vi "ConfigureDlg.vi"(8 "error in (no error)":errorcluster, 11 "PmuTestFunctions in":refnum<class "PmuTestFunctions.lvclass">) -> (0 "error out":errorcluster, 2 "Changed":bool, 3 "PmuTestFunctions out":refnum<class "PmuTestFunctions.lvclass">)   [LabVIEW 2018, in "Functions.lvlib" / "PmuTestFunctions.lvclass"]
uses:
  PmuTestFunctions.lvclass
  X:/Projects/PMUCal/Modules/FGen/MemberClasses/ArbitraryFunction/ArbitraryFunction.lvclass
  X:/Projects/PMUCal/Modules/FGen/MemberClasses/FunctionBaseClass/FunctionBase.lvclass
  ArbitraryFunction/TypeDefs/Arbs.ctl
  Typedefs/PmuTestParams.ctl
  ArbitraryFunction/ArbitraryFunction.lvclass/ArbitraryFunction.ctl
  PmuTestFunctions.lvclass/PmuTestFunctions.ctl
  FunctionBaseClass/FunctionBase.lvclass/FunctionBase.ctl
  ArbitraryFunction/TypeDefs/Arbitrary.ctl
  ArbitraryFunction/Accessors/Read SampleRate.vi
  Accessors/Read PmuTestParams.vi
  Accessors/Read T0.vi
  ArbitraryFunction/Accessors/Read Arbs.vi
  Accessors/Read SettlingTime.vi
  FunctionBaseClass/Accessors/Read FunctionIniFilePath.vi
  ArbitraryFunction/Accessors/Write SampleRate.vi
  Accessors/Write PmuTestParams.vi
  ArbitraryFunction/Accessors/Write Arbs.vi
  ArbitraryFunction/Accessors/Write Count.vi
  Accessors/Write SettlingTime.vi
  FunctionBaseClass/Accessors/Write FunctionIniFilePath.vi
  <vilib>/Utility/config.llb/NI_LVConfig.lvlib
  ArbitraryFunction/ArbitraryFunction.lvclass
panel:
  in  "btnSaveAs":bool
  in  "SettlingTime":dbl
  in  "T0":dbl
  in  "btnSave":bool
  in  "btnCancel":bool
  in  "SampleRate":dbl
  in  "PmuTestParams":T1
  in  "ARBS":T2[](array[typedef])
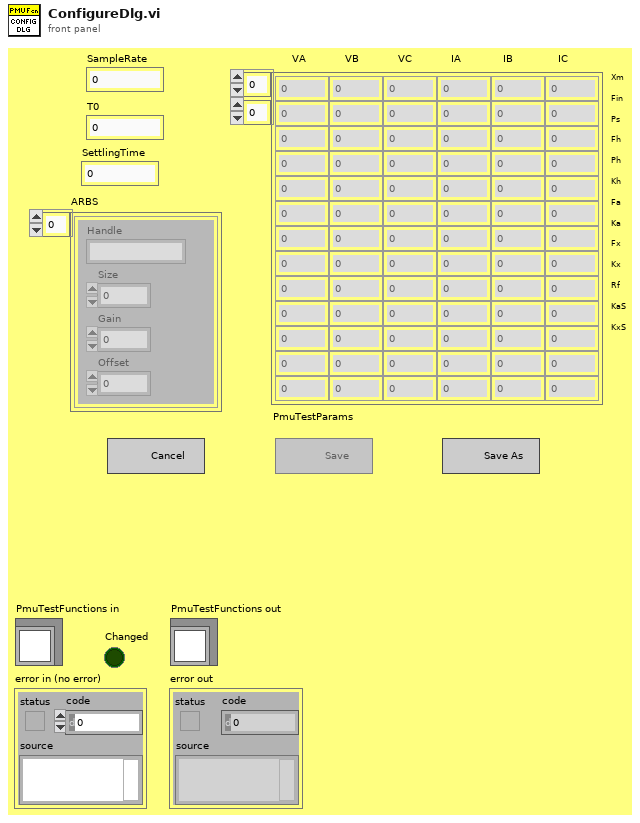
[diagram p1: front panel]
types:
  T1 = typedef "Functions.lvlib/PmuTestFunctions.lvclass/PmuTestParams.ctl" = dbl[][]
  T2 = typedef "Functions.lvlib/ArbitraryFunction.lvclass/Arbs.ctl" = cluster{"Handle":string, "Size":i32, "Gain":dbl, "Offset":dbl}
  T3 = enum32{"Invalid", "Standard", "Closed", "Hidden", "Minimized", "Maximized"}
  T4 = enum32{"Invalid", "Default", "Floating", "Floating/Auto-Hide", "Modal"}
  T5 = enum8{"Enabled", "Disabled", "Disabled and Grayed Out"}
  T6 = cluster{"Handle":string, "Size":i32, "Gain":dbl, "Offset":dbl}
  T7 = typedef "Functions.lvlib/ArbitraryFunction.lvclass/Arbitrary.ctl" = cluster{"Handle":string, "Size":i32, "Gain":dbl, "Offset":dbl, "Waveform":waveform(dbl)}
  T8 = typedef "NI_LVConfig.lvlib/Config Data RefNum.ctl" = refnum<k1>
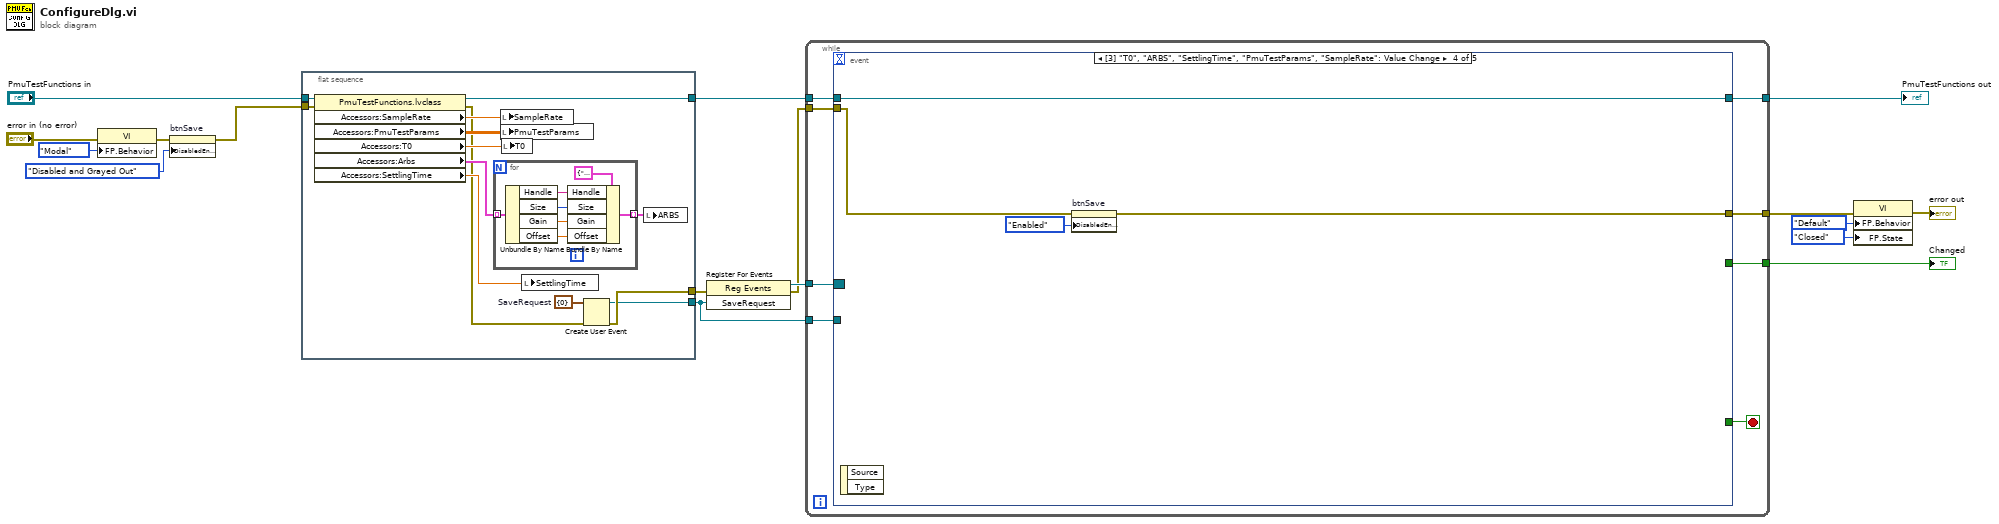
[diagram p0: block diagram]
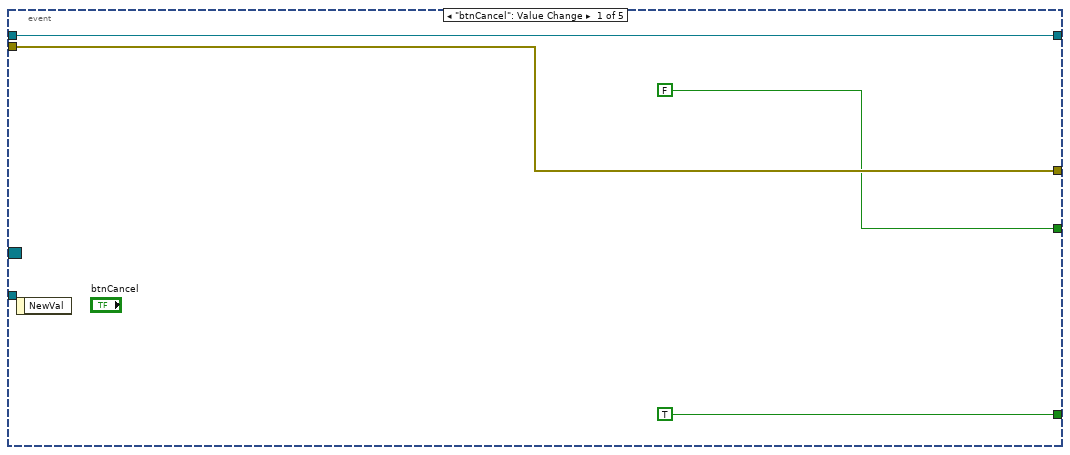
[diagram p2: hidden frame]
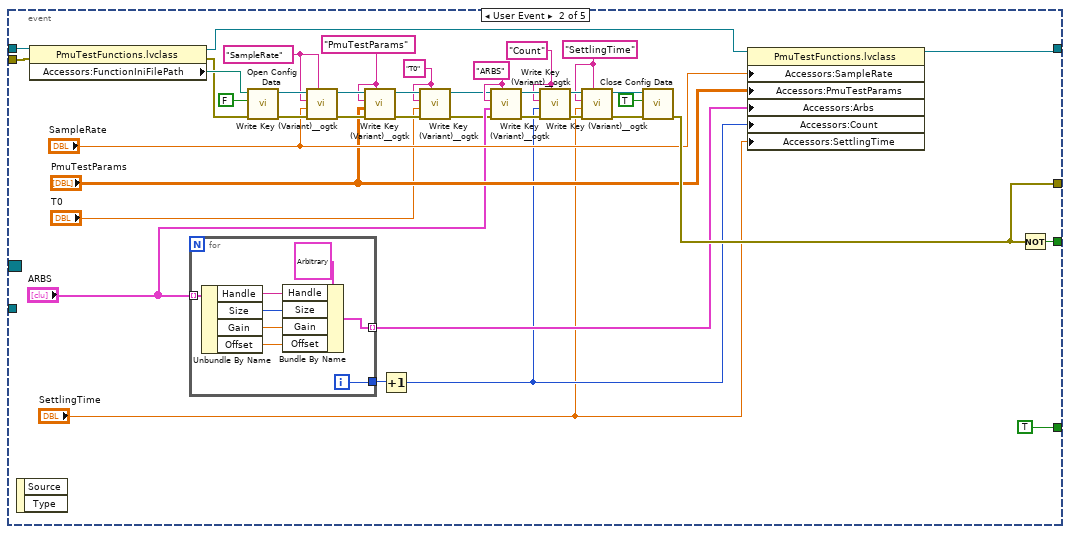
[diagram p3: hidden frame]
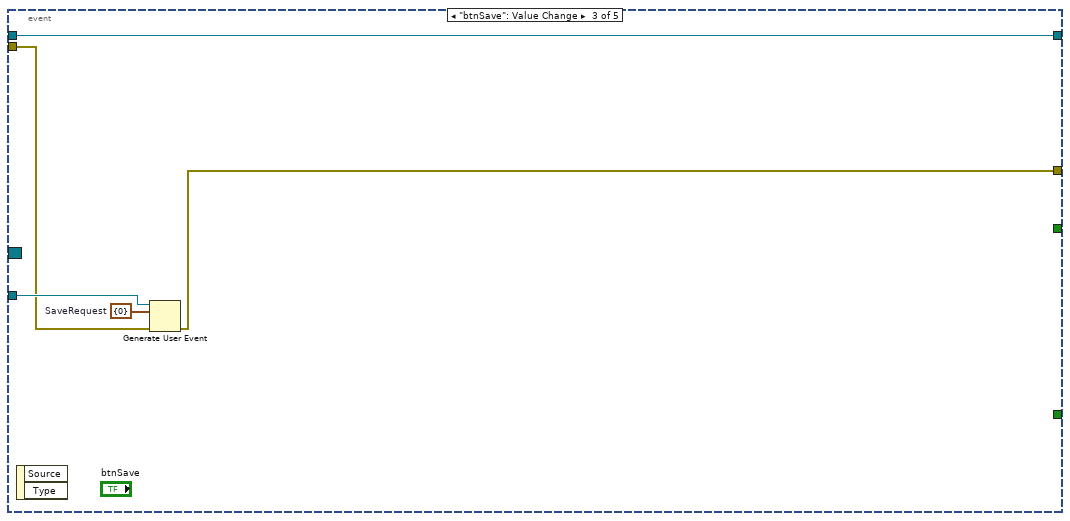
[diagram p4: hidden frame]
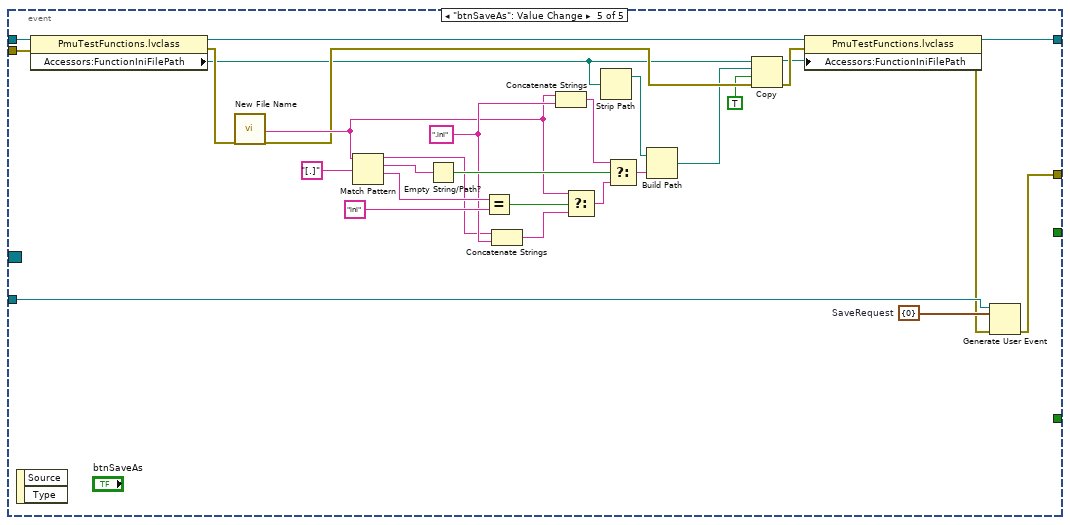
[diagram p5: hidden frame]
diagram:
  n1 = property class="VI"(error in="error in (no error)", "FP.Behavior"=T4."Modal" ("Front Panel Window:Behavior")) -> (error out=w5:errorcluster)  [unwired: 1 in, 1 out]
  n2 = property on="btnSave" class="Bool"(error in=w5, "DisabledEnum"=T5."Disabled and Grayed Out" ("Disabled")) -> (error out=w12:errorcluster)  [unwired: 1 in, 1 out]
  n3 = flat-sequence {
    tunnel: "PmuTestFunctions in" -> [w30]
    tunnel: [w29] -> w16
    tunnel: w12 -> [w27]
    tunnel: [w19] -> w11
    tunnel: [w18] -> w9
    frame #0 {
      w21 = cluster{"num":i32} {"num"=0}  # SaveRequest
      n4 = property class="PmuTestFunctions.lvclass"(reference=w30, error in=w27) -> (reference out=w29:refnum<class "PmuTestFunctions.lvclass">, error out=w20:errorcluster, "Accessors:SampleRate"=w26:dbl, "Accessors:PmuTestParams"=w25:T1, "Accessors:T0"=w24:dbl, "Accessors:Arbs"=w28:T7[], "Accessors:SettlingTime"=w22:dbl)
      n5 = for {
        tunnel: w28 -> [w37] mode=indexing
        tunnel: [w31] -> w23 mode=indexing
        n6 = Unbundle By Name(w37) -> ("Handle"=w35:string, "Size"=w34:i32, "Gain"=w33:dbl, "Offset"=w32:dbl)
        n7 = Bundle By Name(cluster=T6 {"Handle"="", "Size"=0, "Gain"=0.0, "Offset"=0.0} ("Arbs"), "Handle"=w35, "Size"=w34, "Gain"=w33, "Offset"=w32) -> (w31:T6)
      }
      n8 = local write "SampleRate"(w26) -> ()
      n9 = local write "PmuTestParams"(w25) -> ()
      n10 = local write "T0"(w24) -> ()
      n11 = local write "SettlingTime"(w22) -> ()
      n12 = Create User Event(user event datatype=w21, error in=w20) -> (user event=w18:refnum<user-event>, error out=w19:errorcluster)
      n13 = local write "ARBS"(w23) -> ()
    }
  }
  n14 = register-events(error in=w11, w9) -> (reference out=w10:refnum<event-registration>, error out=w8:errorcluster)  [unwired: 1 in]
  n15 = while {
    tunnel: w16 -> [w43]
    tunnel: w8 -> [w45]
    tunnel: [w44] -> w3
    tunnel: [w42] -> w15
    tunnel: [w41] -> w14
    tunnel: w10 -> [w39]
    tunnel: w9 -> [w38]
    stop <- w40 stop-if-true
    n16 = event shown="[3] \"T0\", \"ARBS\", \"SettlingTime\", \"PmuTestParams\", \"SampleRate\": Value Change" {
      selector: w39 -> [_ _ _ _ _]
      dyn-events: _ -> [_ _ _ _ _]
      timeout: _ -> [_ _ _ _ _]
      tunnel: [w49 w71 w98 w102 w113] -> w44
      tunnel: w45 -> [w49 w84 w99 w104 w119]
      tunnel: w43 -> [w48 w88 w97 w105 w121]
      tunnel: [w48 w65 w97 w105 w117] -> w42
      tunnel: [FALSE w72 _ _ _] -> w41
      tunnel: [TRUE TRUE _ _ _] -> w40
      tunnel: w38 -> [_ _ w100 _ w115]
      event "btnCancel": Value Change {
        n17 = event-data() -> ()  [unwired: 1 in, 1 out]
      }
      event User Event {
        w53 = "SettlingTime" ("section")
        w59 = "T0" ("section")
        w74 = "Count" ("section")
        w63 = "ARBS" ("section (optional)")
        w77 = "PmuTestParams" ("section")
        w81 = "SampleRate" ("section")
        n18 = event-data() -> ()  [unwired: 1 in, 2 out]
        n19 = property class="PmuTestFunctions.lvclass"(reference=w88, error in=w84) -> (reference out=w70:refnum<class "PmuTestFunctions.lvclass">, error out=w83:errorcluster, "Accessors:FunctionIniFilePath"=w87:path)
        n20 = for {
          tunnel: "ARBS" -> [w95] mode=indexing
          tunnel: [w90] -> w67 mode=indexing
          tunnel: [w89] -> w85
          i -> [w89]
          n21 = Unbundle By Name(w95) -> ("Handle"=w94:string, "Size"=w91:i32, "Gain"=w92:dbl, "Offset"=w93:dbl)
          n22 = Bundle By Name(cluster=T7 {"Handle"="", "Size"=0, "Gain"=0.0, "Offset"=0.0, "Waveform"={"t0"=timestamp(0 s since 1904-01-01), "dt"=1.0, "Y"=[]}} ("Arbitrary"), "Handle"=w94, "Size"=w91, "Gain"=w92, "Offset"=w93) -> (w90:T7)
        }
        n23 = call <vilib>:"Open Config Data.vi"("error in (no error)"=w83, "create file if necessary (T)"=FALSE, "configuration file path"=w87) -> ("error out"=w80:errorcluster, "refnum"=w82:T8)  [unwired: 6 in, 1 out]
        n24 = call <userlib>:"Write Key (Variant)__ogtk.vi"("section"=w81, "error in (no error)"=w80, "key-value"="SampleRate", "key (optional)"=w81, "refnum"=w82) -> ("error out"=w79:errorcluster, "refnum out"=w78:T8)  [unwired: 5 in]
        n25 = call <userlib>:"Write Key (Variant)__ogtk.vi"("section"=w77, "error in (no error)"=w79, "key-value"="PmuTestParams", "key (optional)"=w77, "refnum"=w78) -> ("error out"=w61:errorcluster, "refnum out"=w60:T8)  [unwired: 5 in]
        n26 = Increment(x=w85) -> (x+1=w66:i32)
        n27 = call <userlib>:"Write Key (Variant)__ogtk.vi"("section"=w59, "error in (no error)"=w61, "key-value"="T0", "key (optional)"=w59, "refnum"=w60) -> ("error out"=w58:errorcluster, "refnum out"=w57:T8)  [unwired: 5 in]
        n28 = call <userlib>:"Write Key (Variant)__ogtk.vi"("section"=w63, "error in (no error)"=w58, "key-value"="ARBS", "key (optional)"=w63, "refnum"=w57) -> ("error out"=w76:errorcluster, "refnum out"=w75:T8)  [unwired: 5 in]
        n29 = call <userlib>:"Write Key (Variant)__ogtk.vi"("section"=w74, "error in (no error)"=w76, "key-value"=w66, "key (optional)"=w74, "refnum"=w75) -> ("error out"=w55:errorcluster, "refnum out"=w54:T8)  [unwired: 5 in]
        n30 = call <userlib>:"Write Key (Variant)__ogtk.vi"("section"=w53, "error in (no error)"=w55, "key-value"="SettlingTime", "key (optional)"=w53, "refnum"=w54) -> ("error out"=w51:errorcluster, "refnum out"=w52:T8)  [unwired: 5 in]
        n31 = call <vilib>:"Close Config Data.vi"("error in (no error)"=w51, "write file if changed (T)"=TRUE, "refnum"=w52) -> ("error out"=w71:errorcluster)  [unwired: 7 in, 1 out]
        n32 = property class="PmuTestFunctions.lvclass"(reference=w70, "Accessors:SampleRate"="SampleRate", "Accessors:PmuTestParams"="PmuTestParams", "Accessors:Arbs"=w67, "Accessors:Count"=w66, "Accessors:SettlingTime"="SettlingTime") -> (reference out=w65:refnum<class "PmuTestFunctions.lvclass">)  [unwired: 1 in, 1 out]
        n33 = Not(x=w71) -> (.not. x?=w72:bool)
      }
      event "btnSave": Value Change {
        w101 = cluster{"num":i32} {"num"=0}  # SaveRequest
        n34 = event-data() -> ()  [unwired: 1 in, 2 out]
        n35 = Generate User Event(user event=w100, event data cluster=w101, error in=w99) -> (error out=w98:errorcluster)  [unwired: 1 in, 1 out]
      }
      event "T0", "ARBS", "SettlingTime", "SampleRate": Value Change {
        n36 = event-data() -> ()  [unwired: 1 in, 2 out]
        n37 = property on="btnSave" class="Bool"(error in=w104, "DisabledEnum"=T5."Enabled" ("Disabled")) -> (error out=w102:errorcluster)  [unwired: 1 in, 1 out]
      }
      event "btnSaveAs": Value Change {
        w116 = cluster{"num":i32} {"num"=0}  # SaveRequest
        w125 = ".ini" ("string")
        n38 = event-data() -> ()  [unwired: 1 in, 2 out]
        n39 = property class="PmuTestFunctions.lvclass"(reference=w121, error in=w119) -> (reference out=w120:refnum<class "PmuTestFunctions.lvclass">, error out=w118:errorcluster, "Accessors:FunctionIniFilePath"=w110:path)
        n40 = call "New File Name"("error in (no error)"=w118) -> ("File Name"=w122:string, "error out"=w112:errorcluster)  [unwired: 16 in, 1 out]
        n41 = Match Pattern(string=w122, regular expression="[.]" ("string")) -> (before substring=w124:string, match substring=w128:string, after substring=w127:string)  [unwired: 1 in, 1 out]
        n42 = Empty String/Path?(string/path=w128) -> (empty?=w133:bool)
        n43 = Equal?(x=w127, y="ini" ("string")) -> (x = y?=w131:bool)
        n44 = Concatenate Strings(w124, w125) -> (w123:string)
        n45 = Concatenate Strings(w122, w125) -> (w132:string)
        n46 = Select(t=w122, s=w131, f=w123) -> (s? t:f=w130:string)
        n47 = Strip Path(path=w110) -> (stripped path=w109:path)  [unwired: 1 out]
        n48 = Select(t=w132, s=w133, f=w130) -> (s? t:f=w134:string)
        n49 = Build Path(base path=w109, name or relative path=w134) -> (appended path=w107:path)
        n50 = Copy(8:w112, 9:TRUE ("overwrite (F)"), 10:w107, 11:w110) -> (0:w111:errorcluster, 3:w106:path)  [unwired: 1 in, 1 out]
        n51 = property class="PmuTestFunctions.lvclass"(reference=w120, error in=w111, "Accessors:FunctionIniFilePath"=w106) -> (reference out=w117:refnum<class "PmuTestFunctions.lvclass">, error out=w114:errorcluster)
        n52 = Generate User Event(user event=w115, event data cluster=w116, error in=w114) -> (error out=w113:errorcluster)  [unwired: 1 in, 1 out]
      }
    }
  }
  "PmuTestFunctions out" <- w15
  "Changed" <- w14
  n53 = property class="VI"(error in=w3, "FP.Behavior"=T4."Default" ("Front Panel Window:Behavior"), "FP.State"=T3."Closed" ("Front Panel Window:State")) -> (error out=→"error out":errorcluster)  [unwired: 1 in, 1 out]
